vi "graph temp and power.vi"(7 "T cont":T1 {"utility"."therm volt" format="%_6g"; "T status"."Temp" format="%_6g"}) -> (2 "meas index":i32, 8 "T plot":cluster{"t hist":dbl[], "T hist":dbl[]}, 13 "T status.Temp":dbl)   [LabVIEW 2019]
doc: "This subVI manages the data extraction for the time, and temperature for the full history graph in the thermistor experiment. \n\n\nPaul K Dixon\nP3600\nCSUSB Physics"
uses:
  typedefs/temp cont cluster.ctl
  typedefs/temp exec cluster.ctl
  typedefs/temp mode enum.ctl
  typedefs/temp indicator.ctl
  typedefs/temp cont utility.ctl
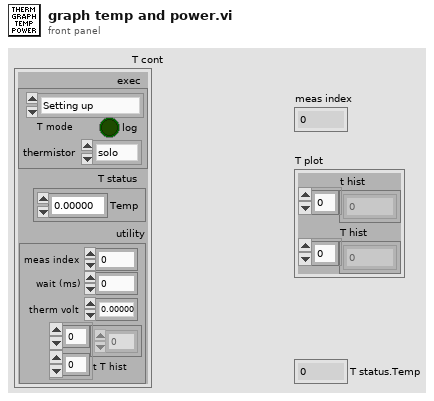
[diagram p1: front panel]
types:
  T1 = typedef "temp cont cluster.ctl" = cluster{"exec":T2, "T status":T4, "utility":T5}
  T2 = typedef "temp exec cluster.ctl" = cluster{"T mode":T3, "log":bool, "thermistor":enum16{"solo", "bug"}}
  T3 = typedef "temp mode enum.ctl" = enum16{"Setting up", "Listening to exec", "Exit"}
  T4 = typedef "temp indicator.ctl" = cluster{"Temp":dbl}
  T5 = typedef "temp cont utility.ctl" = cluster{"meas index":i32, "wait (ms)":i32, "therm volt":dbl, "t T hist":dbl[][]}
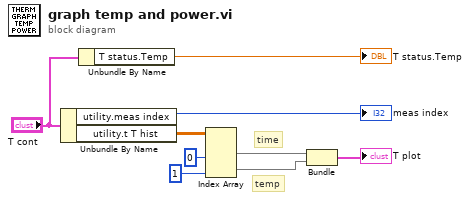
[diagram p0: block diagram]
diagram:
  # "temp"
  # "time"
  n1 = Unbundle By Name("T cont") -> ("utility.meas index"=→"meas index":i32, "utility.t T hist"=w9:dbl[][])
  n2 = Unbundle By Name("T cont") -> ("T status.Temp"=→"T status.Temp":dbl)
  n3 = Index Array(array=w9, index (col) #1=0 ("disabled index (col)"), index (col) #2=1 ("index (col)")) -> (element #1=w7:dbl[], element #2=w8:dbl[])  [unwired: 2 in]
  n4 = Bundle("t T hist"=w7, "t T hist"=w8) -> (→"T plot":cluster{"t T hist":dbl[], "t T hist":dbl[]})  [unwired: 1 in]
